vi "Robot_Track.vi"() -> ()   [LabVIEW 2013]
panel:
  in  "Display History":bool=TRUE
  out "Extra Recieve 1":dbl=255.0
  out "Extra Recieve 2":dbl=255.0
  out "Y Robot":dbl
  in  "Y Offset":dbl=14.0 format="%#_13g"
  in  "X Offset":dbl=8.0 format="%#_13g"
  out "X Robot":dbl
  in  "Stop Button":bool
  in  "Send Data to Robot":bool
  in  "Input 1":dbl
  in  "Input 2":dbl
  out "Robot Map":picture
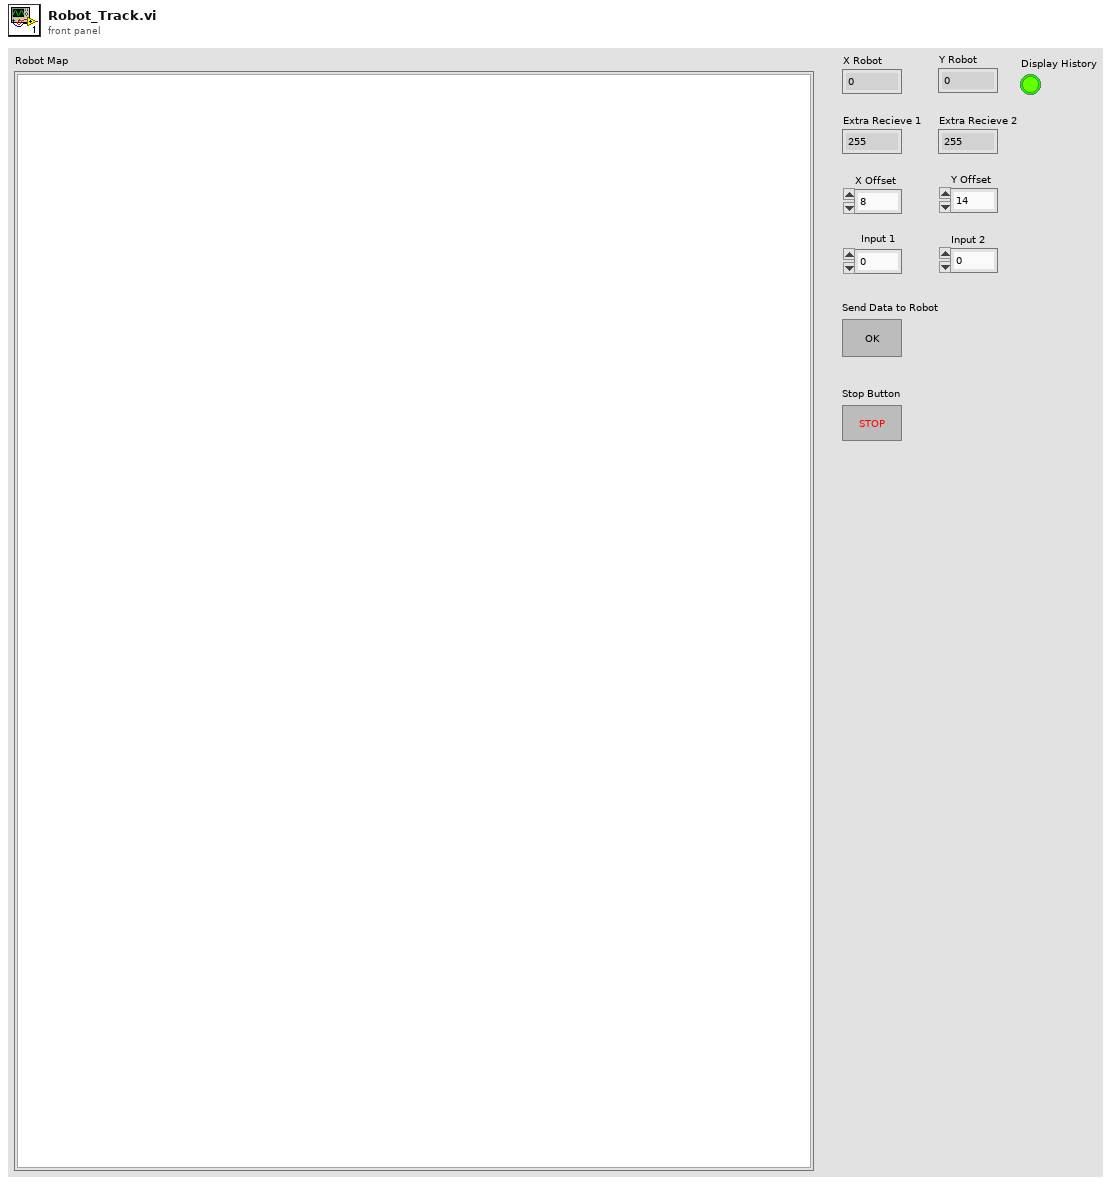
[diagram p1: front panel]
types:
  T1 = enum16{"Standard", "Buffered", "CRLF", "Immediate"}
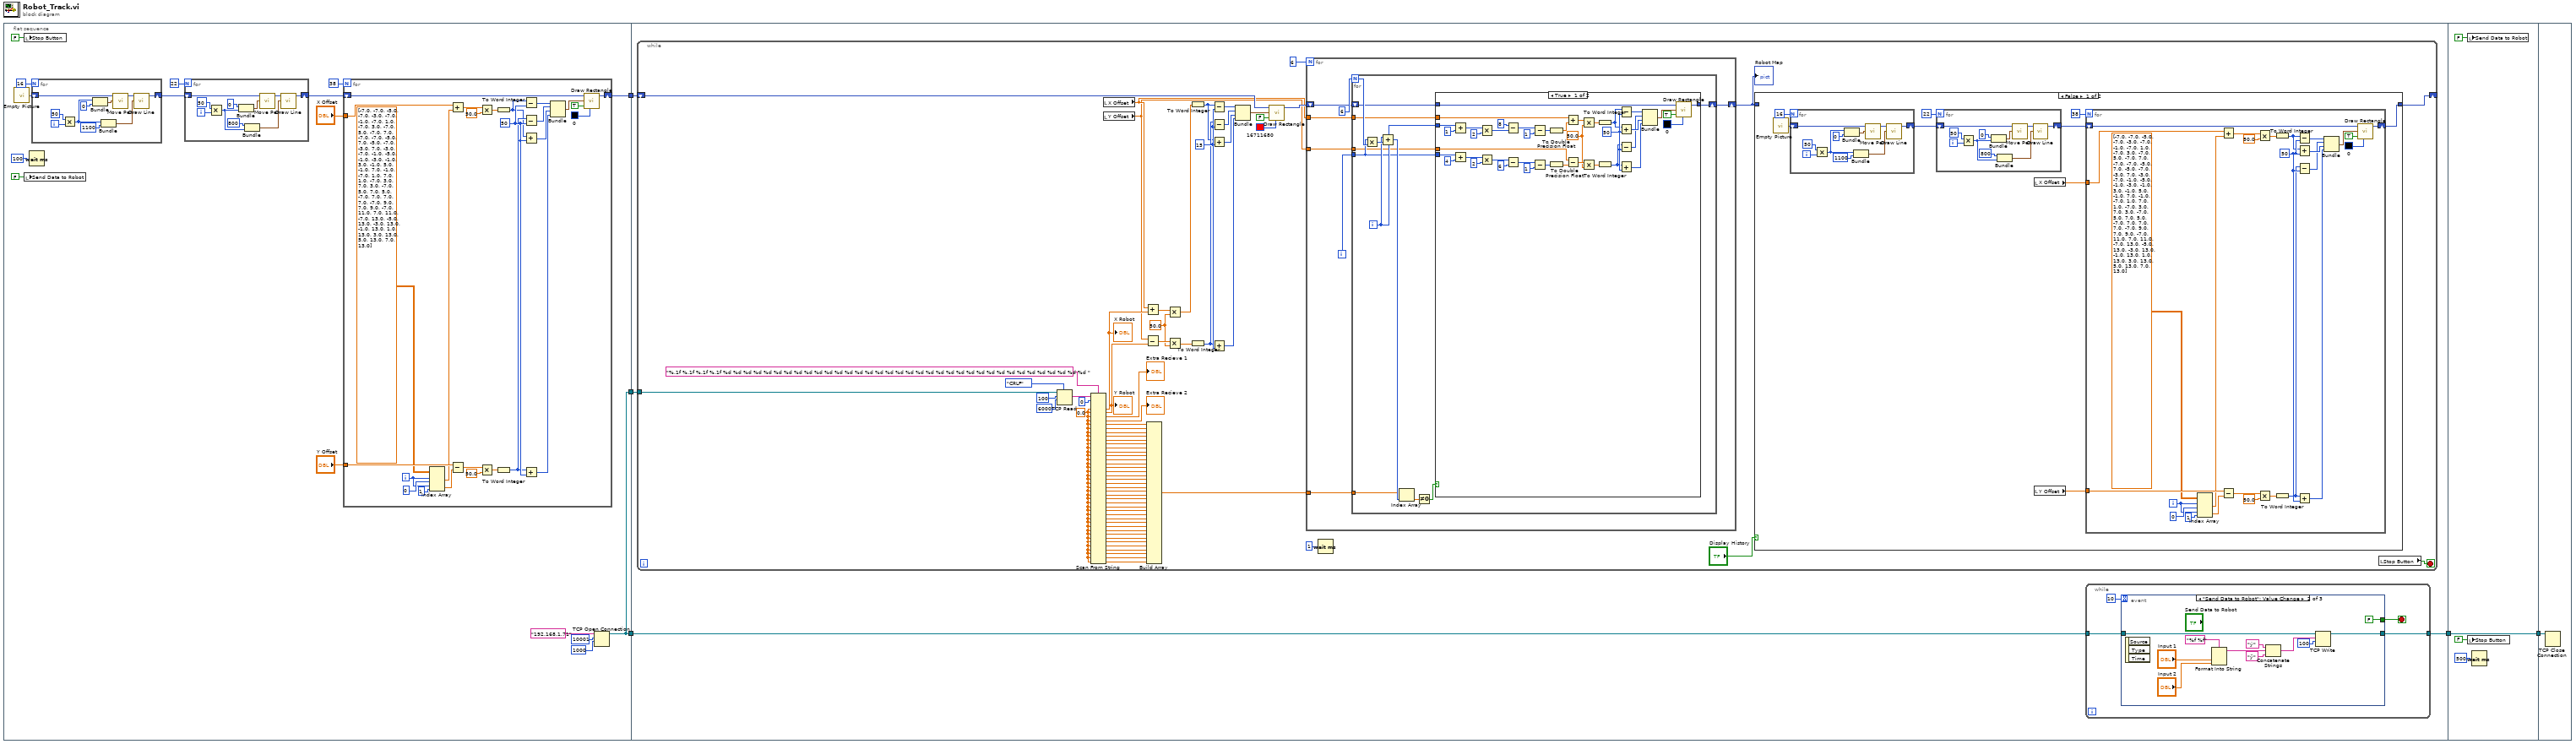
[diagram p0: block diagram]
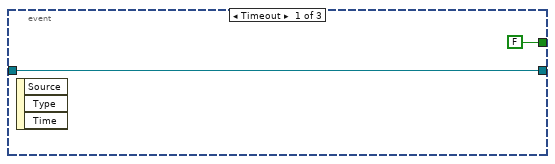
[diagram p4: hidden frame]
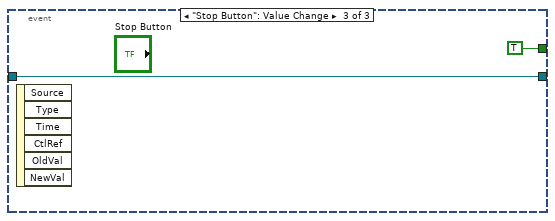
[diagram p5: hidden frame]
diagram:
  n1 = flat-sequence {
    tunnel: [w17] -> w5
    tunnel: [w17] -> w4
    tunnel: [w6] -> w1
    tunnel: w5 -> [w71]
    tunnel: w4 -> [w69]
    tunnel: [w70] -> w3
    tunnel: w1 -> [w68]
    tunnel: w3 -> [w282]
    tunnel: [w282] -> w2
    tunnel: w2 -> [w284]
    frame #0 {
      n2 = call "Empty Picture"() -> ("empty picture"=w14:picture)
      n3 = local write "Stop Button"(FALSE ("stop")) -> ()
      n4 = local write "Send Data to Robot"(FALSE) -> ()
      n5 = Wait (ms)(milliseconds to wait=u32 100) -> ()  [unwired: 1 out]
      n6 = for {
        N: 16 -> [_]
        shift-right: [w59] -> w13
        shift-left: w14 -> [w61]
        i -> [w58]
        n7 = Multiply(x=50, y=w58) -> (x*y=w60:i32)
        n8 = Bundle(w60, i16 0) -> (w63:cluster{i32, i16})  [unwired: 1 in]
        n9 = Bundle(w60, i16 1100) -> (w66:cluster{i32, i16})  [unwired: 1 in]
        n10 = call <vilib>:"Move Pen.vi"("new position"=w63, "picture"=w61) -> ("new picture"=w64:picture)  [unwired: 3 in]
        n11 = call <vilib>:"Draw Line.vi"("picture"=w64, "end point"=w66) -> ("new picture"=w59:picture)  [unwired: 7 in]
      }
      n12 = for {
        N: 22 -> [_]
        shift-right: [w48] -> w7
        shift-left: w13 -> [w50]
        i -> [w49]
        n13 = Multiply(x=50, y=w49) -> (x*y=w53:i32)
        n14 = Bundle(i16 0, w53) -> (w51:cluster{i16, i32})  [unwired: 1 in]
        n15 = Bundle(i16 800, w53) -> (w52:cluster{i16, i32})  [unwired: 1 in]
        n16 = call <vilib>:"Move Pen.vi"("new position"=w51, "picture"=w50) -> ("new picture"=w56:picture)  [unwired: 3 in]
        n17 = call <vilib>:"Draw Line.vi"("picture"=w56, "end point"=w52) -> ("new picture"=w48:picture)  [unwired: 7 in]
      }
      n18 = for {
        N: 38 -> [_]
        tunnel: "X Offset" -> [w28]
        tunnel: "Y Offset" -> [w29]
        shift-right: [w31] -> w6
        shift-left: w7 -> [w32]
        i -> [w25]
        w44 = i16 50 ("Size of Rectangle")
        n19 = Index Array(array=dbl[][] [[-7.0, -7.0], [-5.0, -7.0], [-3.0, -7.0], [-1.0, -7.0], [1.0, -7.0], [3.0, -7.0], [5.0, -7.0], [7.0, -7.0], [-7.0, -5.0], [7.0, -5.0], [-7.0, -3.0], [7.0, -3.0], [-7.0, -1.0], [-5.0, -1.0], [-3.0, -1.0], [3.0, -1.0], [5.0, -1.0], [7.0, -1.0], [-7.0, 1.0], [7.0, 1.0], [-7.0, 3.0], [7.0, 3.0], [-7.0, 5.0], [7.0, 5.0], [-7.0, 7.0], [7.0, 7.0], [-7.0, 9.0], [7.0, 9.0], [-7.0, 11.0], [7.0, 11.0], [-7.0, 13.0], [-5.0, 13.0], [-3.0, 13.0], [-1.0, 13.0], [1.0, 13.0], [3.0, 13.0], [5.0, 13.0], [7.0, 13.0]], index (row) #1=w25, index (col) #1=0 ("disabled index (col)"), index (row) #2=w25, index (col) #2=1 ("disabled index (col)")) -> (element #1=w23:dbl, element #2=w22:dbl)
        n20 = Add(x=w28, y=w23) -> (x+y=w35:dbl)
        n21 = Subtract(x=w29, y=w22) -> (x-y=w34:dbl)
        n22 = Multiply(x=w35, y=50.0) -> (x*y=w37:dbl)
        n23 = Multiply(x=w34, y=50.0) -> (x*y=w45:dbl)
        n24 = To Word Integer(number=w37) -> (16bit integer=w30:i16)
        n25 = To Word Integer(number=w45) -> (16bit integer=w36:i16)
        n26 = Subtract(x=w30, y=w44) -> (x-y=w43:i16)
        n27 = Subtract(x=w36, y=w44) -> (x-y=w41:i16)
        n28 = Add(x=w30, y=w44) -> (x+y=w42:i16)
        n29 = Add(x=w36, y=w44) -> (x+y=w40:i16)
        n30 = Bundle(w43, w41, w42, w40) -> (w39:cluster{i16, i16, i16, i16})  [unwired: 1 in]
        n31 = call <vilib>:"Draw Rectangle.vi"("picture"=w32, "rect"=w39, "fill?(F)"=TRUE, "color(black)"=u32 0) -> ("new picture"=w31:picture)  [unwired: 5 in]
      }
      n32 = TCP Open Connection(address="192.168.1.71", remote port or service name=u16 10001, timeout ms (60000)=1000) -> (connection ID=w17:refnum<k5>)  [unwired: 2 in, 1 out]
    }
    frame #1 {
      n33 = while {
        shift-right: [w72] -> _
        shift-left: w68 -> [w135]
        tunnel: w69 -> [w85]
        stop <- w136 stop-if-true
        w128 = 0.0 ("default value 1")
        w143 = i16 15 ("Size of Rectangle")
        w77 = 50.0 ("y")
        n34 = TCP Read(connection ID=w85, bytes to read=100, 7:T1."CRLF" ("mode (standard)"), 9:6000 ("timeout ms (25000)")) -> (data out=w91:string)  [unwired: 1 in, 2 out]
        n35 = Scan From String(format string="%.1f %.1f %.1f %.1f %d %d %d %d %d %d %d %d %d %d %d %d %d %d %d %d %d %d %d %d %d %d %d %d %d %d %d %d %d %d %d %d %d %d %d %d ", input string=w91, initial scan location=u32 0, default 1=w128, default 2=w128, default 3=w128, default 4=w128, default 5=w128, default 6=w128, default 7=w128, default 8=w128, default 9=w128, default 10=w128, default 11=w128, default 12=w128, default 13=w128, default 14=w128, default 15=w128, default 16=w128, default 17=w128, default 18=w128, default 19=w128, default 20=w128, default 21=w128, default 22=w128, default 23=w128, default 24=w128, default 25=w128, default 26=w128, default 27=w128, default 28=w128, default 29=w128, default 30=w128, default 31=w128, default 32=w128, default 33=w128, default 34=w128, default 35=w128, default 36=w128, default 37=w128, default 38=w128, default 39=w128, default 40=w128) -> (output 1=w80:dbl, output 2=w81:dbl, output 3=→"Extra Recieve 1":dbl, output 4=→"Extra Recieve 2":dbl, output 5=w92:dbl, output 6=w93:dbl, output 7=w94:dbl, output 8=w95:dbl, output 9=w96:dbl, output 10=w97:dbl, output 11=w98:dbl, output 12=w99:dbl, output 13=w100:dbl, output 14=w101:dbl, output 15=w102:dbl, output 16=w103:dbl, output 17=w104:dbl, output 18=w105:dbl, output 19=w106:dbl, output 20=w107:dbl, output 21=w108:dbl, output 22=w109:dbl, output 23=w110:dbl, output 24=w111:dbl, output 25=w112:dbl, output 26=w113:dbl, output 27=w114:dbl, output 28=w115:dbl, output 29=w116:dbl, output 30=w117:dbl, output 31=w118:dbl, output 32=w119:dbl, output 33=w120:dbl, output 34=w121:dbl, output 35=w122:dbl, output 36=w123:dbl, output 37=w124:dbl, output 38=w125:dbl, output 39=w126:dbl, output 40=w127:dbl)  [unwired: 1 in, 3 out]
        "X Robot" <- w80
        "Y Robot" <- w81
        n36 = local read "X Offset"() -> (w79:dbl)
        n37 = local read "Y Offset"() -> (w78:dbl)
        n38 = Add(x=w79, y=w80) -> (x+y=w131:dbl)
        n39 = Subtract(x=w78, y=w81) -> (x-y=w130:dbl)
        n40 = Build Array(w92, w93, w94, w95, w96, w97, w98, w99, w100, w101, w102, w103, w104, w105, w106, w107, w108, w109, w110, w111, w112, w113, w114, w115, w116, w117, w118, w119, w120, w121, w122, w123, w124, w125, w126, w127) -> (w83:dbl[])
        n41 = Multiply(x=w131, y=w77) -> (x*y=w134:dbl)
        n42 = Multiply(x=w130, y=w77) -> (x*y=w144:dbl)
        n43 = To Word Integer(number=w134) -> (16bit integer=w132:i16)
        n44 = To Word Integer(number=w144) -> (16bit integer=w133:i16)
        n45 = Subtract(x=w132, y=w143) -> (x-y=w142:i16)
        n46 = Subtract(x=w133, y=w143) -> (x-y=w140:i16)
        n47 = Add(x=w132, y=w143) -> (x+y=w141:i16)
        n48 = Add(x=w133, y=w143) -> (x+y=w139:i16)
        n49 = Bundle(w142, w140, w141, w139) -> (w138:cluster{i16, i16, i16, i16})  [unwired: 1 in]
        n50 = call <vilib>:"Draw Rectangle.vi"("picture"=w135, "rect"=w138, "fill?(F)"=FALSE, "color(black)"=u32 16711680) -> ("new picture"=w82:picture)  [unwired: 5 in]
        n51 = for {
          N: 6 -> [_]
          tunnel: w83 -> [w206]
          shift-right: [w205] -> w73
          shift-left: w82 -> [w204]
          tunnel: w79 -> [w203]
          tunnel: w78 -> [w202]
          i -> [w207]
          n52 = for {
            N: 6 -> [w220]
            tunnel: w207 -> [w213]
            tunnel: w206 -> [w217]
            shift-right: [w212] -> w205
            shift-left: w204 -> [w211]
            tunnel: w203 -> [w210]
            tunnel: w202 -> [w209]
            i -> [w214]
            n53 = Multiply(x=w213, y=w220) -> (x*y=w219:i32)
            n54 = Add(x=w214, y=w219) -> (x+y=w218:i32)
            n55 = Index Array(array=w217, index=w218) -> (element=w216:dbl)
            n56 = Not Equal To 0?(x=w216) -> (x != 0?=w215:bool)
            n57 = case shown="True" w215 {
              tunnel: w211 -> [w224 w260]
              tunnel: w214 -> [w246 _]
              tunnel: w213 -> [w249 _]
              tunnel: [w225 w260] -> w212
              tunnel: w210 -> [w243 _]
              tunnel: w209 -> [w242 _]
              frame True {
                w236 = i16 50 ("Size of Rectangle")
                w221 = 50.0 ("y")
                n58 = Add(x=w246, y=1) -> (x+y=w245:i32)
                n59 = Add(x=w249, y=4) -> (x+y=w248:i32)
                n60 = Multiply(x=w245, y=2) -> (x*y=w258:i32)
                n61 = Multiply(x=w248, y=2) -> (x*y=w251:i32)
                n62 = Subtract(x=8, y=w258) -> (x-y=w256:i32)
                n63 = Subtract(x=w251, y=6) -> (x-y=w253:i32)
                n64 = Subtract(x=w256, y=1) -> (x-y=w239:i32)
                n65 = Subtract(x=w253, y=1) -> (x-y=w241:i32)
                n66 = To Double Precision Float(number=w239) -> (double precision float=w238:dbl)
                n67 = To Double Precision Float(number=w241) -> (double precision float=w240:dbl)
                n68 = Add(x=w243, y=w238) -> (x+y=w223:dbl)
                n69 = Subtract(x=w242, y=w240) -> (x-y=w222:dbl)
                n70 = Multiply(x=w223, y=w221) -> (x*y=w229:dbl)
                n71 = Multiply(x=w222, y=w221) -> (x*y=w237:dbl)
                n72 = To Word Integer(number=w229) -> (16bit integer=w227:i16)
                n73 = To Word Integer(number=w237) -> (16bit integer=w228:i16)
                n74 = Subtract(x=w227, y=w236) -> (x-y=w235:i16)
                n75 = Add(x=w227, y=w236) -> (x+y=w234:i16)
                n76 = Subtract(x=w228, y=w236) -> (x-y=w233:i16)
                n77 = Add(x=w228, y=w236) -> (x+y=w232:i16)
                n78 = Bundle(w235, w233, w234, w232) -> (w231:cluster{i16, i16, i16, i16})  [unwired: 1 in]
                n79 = call <vilib>:"Draw Rectangle.vi"("picture"=w224, "rect"=w231, "fill?(F)"=TRUE, "color(black)"=u32 0) -> ("new picture"=w225:picture)  [unwired: 5 in]
              }
              frame False {
              }
            }
          }
        }
        "Robot Map" <- w73
        n80 = Wait (ms)(milliseconds to wait=u32 1) -> ()  [unwired: 1 out]
        n81 = case shown="False" "Display History" {
          tunnel: [w150 w201] -> w72
          tunnel: w73 -> [_ w201]
          frame False {
            n82 = call "Empty Picture"() -> ("empty picture"=w151:picture)
            n83 = for {
              N: 16 -> [_]
              shift-right: [w192] -> w152
              shift-left: w151 -> [w194]
              i -> [w191]
              n84 = Multiply(x=50, y=w191) -> (x*y=w193:i32)
              n85 = Bundle(w193, i16 0) -> (w196:cluster{i32, i16})  [unwired: 1 in]
              n86 = Bundle(w193, i16 1100) -> (w199:cluster{i32, i16})  [unwired: 1 in]
              n87 = call <vilib>:"Move Pen.vi"("new position"=w196, "picture"=w194) -> ("new picture"=w197:picture)  [unwired: 3 in]
              n88 = call <vilib>:"Draw Line.vi"("picture"=w197, "end point"=w199) -> ("new picture"=w192:picture)  [unwired: 7 in]
            }
            n89 = for {
              N: 22 -> [_]
              shift-right: [w181] -> w146
              shift-left: w152 -> [w183]
              i -> [w182]
              n90 = Multiply(x=50, y=w182) -> (x*y=w186:i32)
              n91 = Bundle(i16 0, w186) -> (w184:cluster{i16, i32})  [unwired: 1 in]
              n92 = Bundle(i16 800, w186) -> (w185:cluster{i16, i32})  [unwired: 1 in]
              n93 = call <vilib>:"Move Pen.vi"("new position"=w184, "picture"=w183) -> ("new picture"=w189:picture)  [unwired: 3 in]
              n94 = call <vilib>:"Draw Line.vi"("picture"=w189, "end point"=w185) -> ("new picture"=w181:picture)  [unwired: 7 in]
            }
            n95 = local read "X Offset"() -> (w148:dbl)
            n96 = local read "Y Offset"() -> (w147:dbl)
            n97 = for {
              N: 38 -> [_]
              tunnel: w148 -> [w161]
              tunnel: w147 -> [w162]
              shift-right: [w164] -> w150
              shift-left: w146 -> [w165]
              i -> [w158]
              w177 = i16 50 ("Size of Rectangle")
              n98 = Index Array(array=dbl[][] [[-7.0, -7.0], [-5.0, -7.0], [-3.0, -7.0], [-1.0, -7.0], [1.0, -7.0], [3.0, -7.0], [5.0, -7.0], [7.0, -7.0], [-7.0, -5.0], [7.0, -5.0], [-7.0, -3.0], [7.0, -3.0], [-7.0, -1.0], [-5.0, -1.0], [-3.0, -1.0], [3.0, -1.0], [5.0, -1.0], [7.0, -1.0], [-7.0, 1.0], [7.0, 1.0], [-7.0, 3.0], [7.0, 3.0], [-7.0, 5.0], [7.0, 5.0], [-7.0, 7.0], [7.0, 7.0], [-7.0, 9.0], [7.0, 9.0], [-7.0, 11.0], [7.0, 11.0], [-7.0, 13.0], [-5.0, 13.0], [-3.0, 13.0], [-1.0, 13.0], [1.0, 13.0], [3.0, 13.0], [5.0, 13.0], [7.0, 13.0]], index (row) #1=w158, index (col) #1=0 ("disabled index (col)"), index (row) #2=w158, index (col) #2=1 ("disabled index (col)")) -> (element #1=w156:dbl, element #2=w155:dbl)
              n99 = Add(x=w161, y=w156) -> (x+y=w168:dbl)
              n100 = Subtract(x=w162, y=w155) -> (x-y=w167:dbl)
              n101 = Multiply(x=w168, y=50.0) -> (x*y=w170:dbl)
              n102 = Multiply(x=w167, y=50.0) -> (x*y=w178:dbl)
              n103 = To Word Integer(number=w170) -> (16bit integer=w163:i16)
              n104 = To Word Integer(number=w178) -> (16bit integer=w169:i16)
              n105 = Subtract(x=w163, y=w177) -> (x-y=w176:i16)
              n106 = Add(x=w163, y=w177) -> (x+y=w175:i16)
              n107 = Subtract(x=w169, y=w177) -> (x-y=w174:i16)
              n108 = Add(x=w169, y=w177) -> (x+y=w173:i16)
              n109 = Bundle(w176, w174, w175, w173) -> (w172:cluster{i16, i16, i16, i16})  [unwired: 1 in]
              n110 = call <vilib>:"Draw Rectangle.vi"("picture"=w165, "rect"=w172, "fill?(F)"=TRUE, "color(black)"=u32 0) -> ("new picture"=w164:picture)  [unwired: 5 in]
            }
          }
          frame True {
          }
        }
        n111 = local read "Stop Button"() -> (w136:bool)
      }
      n112 = while {
        tunnel: w71 -> [w263]
        tunnel: [w264] -> w70
        stop <- w261 stop-if-true
        n113 = event shown="[1] \"Send Data to Robot\": Value Change" {
          selector: _ -> [_ _ _]
          dyn-events: _ -> [_ _ _]
          timeout: 10 -> [_ _ _]
          tunnel: [w266 w267 w279] -> w264
          tunnel: w263 -> [w266 w268 w279]
          tunnel: [FALSE FALSE TRUE] -> w261
          event Timeout {
            n114 = event-data() -> ()  [unwired: 1 in, 3 out]
          }
          event "Send Data to Robot": Value Change {
            n115 = event-data() -> ()  [unwired: 1 in, 3 out]
            n116 = Format Into String(format string="%f %f", "Input 1", "Input 2") -> (resulting string=w274:string)  [unwired: 2 in, 1 out]
            n117 = Concatenate Strings("ý" ("string"), w274, "ÿ" ("string")) -> (w269:string)
            n118 = TCP Write(connection ID=w268, data in=w269, 9:100 ("timeout ms (25000)")) -> (connection ID out=w267:refnum<k5>)  [unwired: 1 in, 2 out]
          }
          event "Stop Button": Value Change {
            n119 = event-data() -> ()  [unwired: 1 in, 6 out]
          }
        }
      }
    }
    frame #2 {
      n120 = local write "Send Data to Robot"(FALSE) -> ()
      n121 = local write "Stop Button"(FALSE ("stop")) -> ()
      n122 = Wait (ms)(milliseconds to wait=u32 500) -> ()  [unwired: 1 out]
    }
    frame #3 {
      n123 = TCP Close Connection(connection ID=w284) -> ()  [unwired: 2 in, 2 out]
    }
  }
